vi "MGI Nth Root.vi"(12 "Root":i32=3, 14 "x":dbl format="%.2f") -> (2 "Numeric":dbl format="%.2f")   [LabVIEW 2016]
doc: "Take the nth root of x. Handles x<0 when n is odd, returning the negative real root.\n\nAuthored by David A. Moore\nsupport@mooregoodideas.com\nwww.mooregoodideas.com\n\nCopyright (c) 2010, Moore Good Ideas, Inc.\n\nAll rights reserved.\n\nRedistribution and use in source and binary forms, with or without modification, are permitted provided that the following conditions are met:\n\n * Redistributions of source code must retain the above copyright notice, this list of conditions and the following disclaimer.\n * Redistributions in binary form must reproduce the above copyright notice, this list of conditions and the following disclaimer in the documentation and/or other materials provided with the distribution.\n * Neither the name of Moore Good Ideas, Inc. nor the names of its contributors may be used to endorse or promote products derived from this software without specific prior written permission.\n\nTHIS SOFTWARE IS PROVIDED BY THE COPYRIGHT HOLDERS AND CONTRIBUTORS \"AS IS\" AND ANY EXPRESS OR IMPLIED WARRANTIES, INCLUDING, BUT NOT LIMITED TO, THE IMPLIED WARRANTIES OF MERCHANTABILITY AND FITNESS FOR A PARTICULAR PURPOSE ARE DISCLAIMED. IN NO EVENT SHALL THE COPYRIGHT OWNER OR CONTRIBUTORS BE LIABLE FOR ANY DIRECT, INDIRECT, INCIDENTAL, SPECIAL, EXEMPLARY, OR CONSEQUENTIAL DAMAGES (INCLUDING, BUT NOT LIMITED TO, PROCUREMENT OF SUBSTITUTE GOODS OR SERVICES; LOSS OF USE, DATA, OR PROFITS; OR BUSINESS INTERRUPTION) HOWEVER CAUSED AND ON ANY THEORY OF LIABILITY, WHETHER IN CONTRACT, STRICT LIABILITY, OR TORT (INCLUDING NEGLIGENCE OR OTHERWISE) ARISING IN ANY WAY OUT OF THE USE OF THIS SOFTWARE, EVEN IF ADVISED OF THE POSSIBILITY OF SUCH DAMAGE."
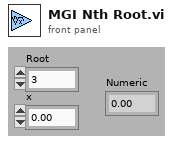
[diagram p1: front panel]
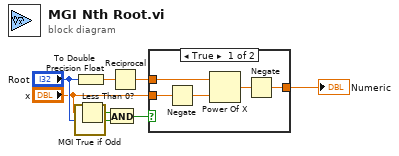
[diagram p0: block diagram]
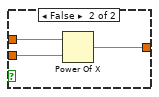
[diagram p2: hidden frame]
diagram:
  n1 = call <userlib>:"MGI True if Odd.vi"("Integer"="Root") -> ("Odd?"=w3:bool)
  n2 = To Double Precision Float(number="Root") -> (double precision float=w7:dbl)
  n3 = Less Than 0?(x="x") -> (x < 0?=w4:bool)
  n4 = And(x=w4, y=w3) -> (x .and. y?=w2:bool)
  n5 = Reciprocal(x=w7) -> (1/x=w8:dbl)
  n6 = case shown="True" w2 {
    tunnel: w8 -> [w13 w16]
    tunnel: "x" -> [w12 w15]
    tunnel: [w9 w14] -> w1
    frame True {
      n7 = Negate(x=w12) -> (-x=w10:dbl)
      n8 = Power Of X(1:w10, 2:w13) -> (0:w11:dbl)
      n9 = Negate(x=w11) -> (-x=w9:dbl)
    }
    frame False {
      n10 = Power Of X(1:w15, 2:w16) -> (0:w14:dbl)
    }
  }
  "Numeric" <- w1
